vi "Populate Commit History Table.vi"(8 "error in":errorcluster, 11 "Peer Review in":refnum<class "Peer Review.lvclass">) -> (0 "error out":errorcluster, 3 "Peer Review out":refnum<class "Peer Review.lvclass">)   [LabVIEW 2020, in "Peer Review.lvclass"]
uses:
  Peer Review.lvclass
  Peer Review.lvclass/Peer Review.ctl
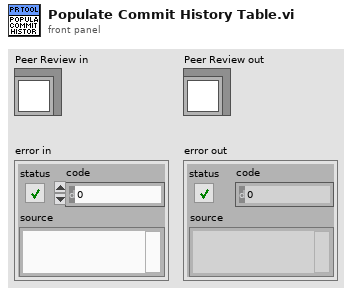
[diagram p1: front panel]
types:
  T1 = typedef "Peer Review.lvclass/Commit Info.ctl" = cluster{"Commit ID":i32, "Hash":string, "Merge Commit?":bool, "Merge Hash":string, "Author":string, "Time Stamp":timestamp, "Description":string, "File Count":i32, "File List":string[]}
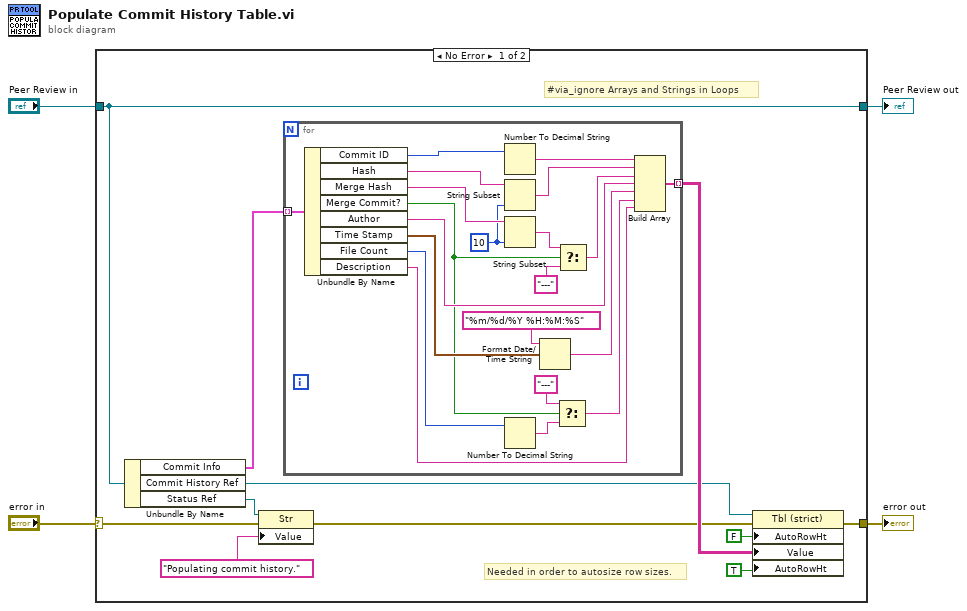
[diagram p0: block diagram]
diagram:
  n1 = case shown="No Error" "error in" {
    selector: "error in" -> [w9 w38]
    tunnel: [w13 w38] -> w4
    tunnel: "Peer Review in" -> [w15 w37]
    tunnel: [w15 w37] -> w1
    frame No Error {
      # "#via_ignore Arrays and Strings in Loops"
      # "Needed in order to autosize row sizes."
      n2 = Unbundle By Name(w15) -> ("Commit Info"=w7:T1[], "Commit History Ref"=w6:refnum<vi>, "Status Ref"=w10:refnum<vi>)
      n3 = property class="Str"(reference=w10, error in=w9, "Value"="Populating commit history.") -> (error out=w8:errorcluster)  [unwired: 1 out]
      n4 = for {
        tunnel: [w36] -> w14 mode=indexing
        tunnel: w7 -> [w35] mode=indexing
        w22 = 10 ("length (rest)")
        n5 = Unbundle By Name(w35) -> ("Commit ID"=w34:i32, "Hash"=w32:string, "Merge Hash"=w29:string, "Merge Commit?"=w20:bool, "Author"=w27:string, "Time Stamp"=w26:timestamp, "File Count"=w21:i32, "Description"=w23:string)
        n6 = Number To Decimal String(number=w34) -> (decimal integer string=w33:string)  [unwired: 1 in]
        n7 = String Subset(string=w32, length (rest)=w22) -> (substring=w31:string)  [unwired: 1 in]
        n8 = String Subset(string=w29, length (rest)=w22) -> (substring=w28:string)  [unwired: 1 in]
        n9 = Number To Decimal String(number=w21) -> (decimal integer string=w19:string)  [unwired: 1 in]
        n10 = Format Date/Time String(time format string (%c)="%m/%d/%Y %H:%M:%S", seconds (now)=w26) -> (date/time string=w24:string)  [unwired: 1 in]
        n11 = Select(t="---", s=w20, f=w19) -> (s? t:f=w18:string)
        n12 = Select(t=w28, s=w20, f="---" ("t")) -> (s? t:f=w30:string)
        n13 = Build Array(w33, w31, w30, w27, w24, w18, w23) -> (w36:string[])
      }
      n14 = property on="Property Node" class="Tbl (strict)"(reference=w6, error in=w8, "AutoRowHt"=FALSE ("Autosizing Row Height"), "Value"=w14, "AutoRowHt"=TRUE ("Autosizing Row Height")) -> (error out=w13:errorcluster)  [unwired: 1 out]
    }
    frame Error {
    }
  }
  "error out" <- w4
  "Peer Review out" <- w1
